vi "901x 9870 DMA Write (Sub).vi"(8 "error in":errorcluster, 10 "Send Data":string) -> (0 "error out":errorcluster, 1 "Byte Count":u32, 4 "Timed Out":bool, 6 "FPGA Error":errorcluster)   [LabVIEW 2012]
uses:
  <vilib>/rvi/interface/nirviMethod/nirviMethod.xnode
  <vilib>/rvi/interface/nirviReadWriteControl/nirviReadWriteControl.xnode
  FPGA Function.ctl
  <vilib>/rvi/errors/niLvFpgaMergeErrorWithErrorCode.vi
  <vilib>/rvi/interface/Simulation/niFpgaSimulationCallBeginRW.vi
  <vilib>/rvi/errors/niLvFpgaAdjustHostInterfaceError.vi
  <vilib>/FPGAPlugInAG/Dynamic/niLvFpga_WriteFifo_Dynamic.vi
  <vilib>/FPGAPlugInAG/Dynamic/niLvFpga_AcknowledgeIrq_Dynamic.vi
  <vilib>/rvi/interface/nirviMethod/StockFPGA_InlinedMethodWaitForSingleIRQ.vi
  <vilib>/FPGAPlugInAG/Dynamic/niLvFpga_WaitOnIrq_Dynamic.vi
panel:
  in  "FPGA Interface":refnum<k20>
  # "INPUTS"
  # "OUTPUTS"
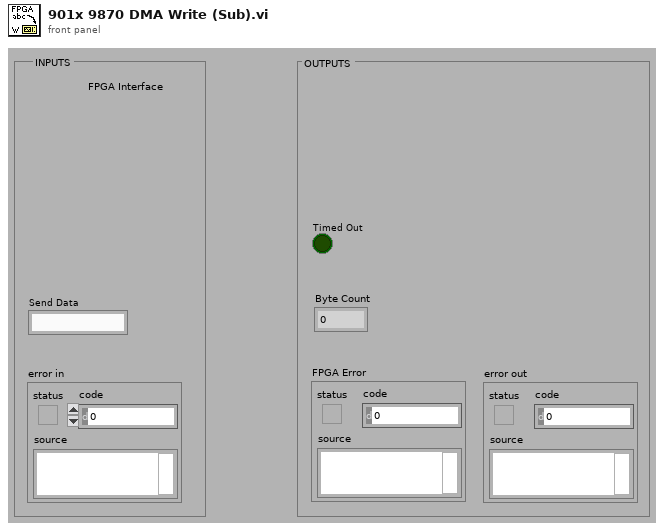
[diagram p1: front panel]
types:
  T1 = typedef "FPGA Function.ctl" = enum16{"Do Nothing", "Write", "Read"}
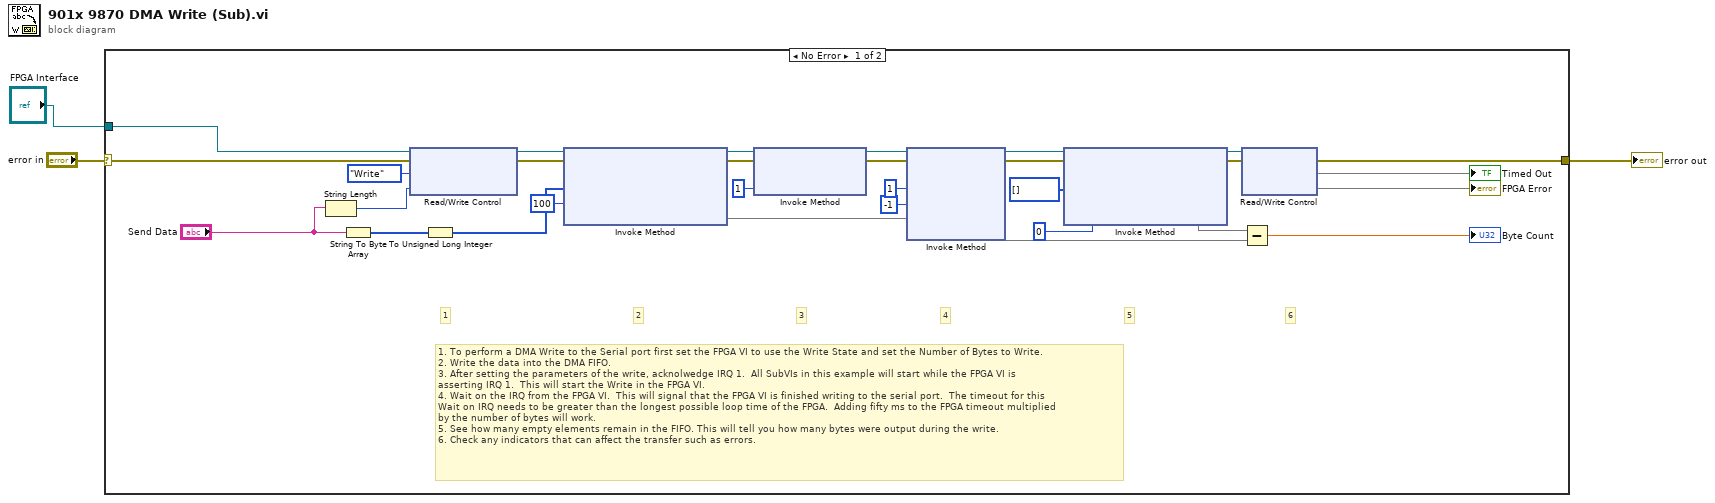
[diagram p0: block diagram]
diagram:
  n1 = case shown="No Error" "error in" {
    selector: "error in" -> [w7 w34]
    tunnel: [w33 w34] -> w3
    tunnel: "FPGA Interface" -> [w4 _]
    frame No Error {
      # "5"
      # "6"
      # "4"
      # "3"
      # "2"
      # "1"
      # "1. To perform a DMA Write to the Serial port first set the FPGA VI to use the Write State and set the Number of Bytes to Write.\n2. Write the data into the DMA FIFO.\n3. After setting the parameters of the write, acknolwedge IRQ 1.  All SubVIs in this example will start while the FPGA VI is \nasserting IRQ 1.  This will start the Write in the FPGA VI.\n4. Wait on the IRQ from the FPGA VI.  This will signal that the FPGA VI is finished writing to the serial port.  The timeout for this \nWait on IRQ needs to be greater than the longest possible loop time of the FPGA.  Adding fifty ms to the FPGA timeout multiplied \nby the number of bytes will work.\n5. See how many empty elements remain in the FIFO. This will tell you how many bytes were output during the write.\n6. Check any indicators that can affect the transfer such as errors."
      n2 = String Length(string="Send Data") -> (length=w6:i32)
      n3 = String To Byte Array(string="Send Data") -> (unsigned byte array=w19:u8[])
      n4 = xnode "Read/Write Control"("FPGA VI Reference In"=w4, "error in"=w7, "Op Control"=FPGA_Function."Write", "Number of Bytes"=w6) -> ("FPGA VI Reference Out"=w31:refnum<k20>, "error out"=w30:errorcluster)
      n5 = To Unsigned Long Integer(number=w19) -> (unsigned 32bit integer=w18:u32[])
      n6 = xnode "Invoke Method"("FPGA VI Reference In"=w31, "error in"=w30, "Data"=w18, "Timeout (ms)"=100) -> ("FPGA VI Reference Out"=w27:refnum<k20>, "error out"=w26:errorcluster, "Empty Elements Remaining"=w9)
      n7 = xnode "Invoke Method"("FPGA VI Reference In"=w27, "error in"=w26, "IRQ Number(s)"=1) -> ("FPGA VI Reference Out"=w25:refnum<k20>, "error out"=w24:errorcluster)
      n8 = xnode "Invoke Method"("FPGA VI Reference In"=w25, "error in"=w24, "IRQ Number(s)"=1, "Timeout (ms)"=-1) -> ("FPGA VI Reference Out"=w16:refnum<k20>, "error out"=w15:errorcluster)  [unwired: 2 out]
      n9 = xnode "Invoke Method"("FPGA VI Reference In"=w16, "error in"=w15, "Data"=u32[] [], "Timeout (ms)"=0) -> ("FPGA VI Reference Out"=w14:refnum<k20>, "error out"=w13:errorcluster, "Empty Elements Remaining"=w10)
      n10 = xnode "Read/Write Control"("FPGA VI Reference In"=w14, "error in"=w13) -> ("FPGA VI Reference Out"=w21:refnum<k20>, "error out"=w33:errorcluster, "Timed Out"=→"Timed Out", "error out"=→"FPGA Error")
      n11 = Subtract(x=w10, y=w9) -> (x-y=→"Byte Count":dbl)
    }
    frame Error {
    }
  }
  "error out" <- w3
